vi "power supply newest.vi"() -> ()   [LabVIEW 2022 SP3]
uses:
  <vilib>/DAQmx/create/channels.llb/DAQmx Create Channel (AI-Voltage-Basic).vi
  <vilib>/DAQmx/read.llb/DAQmx Read (Analog DBL 1Chan 1Samp).vi
panel:
  in  "physical channels":tag
  out "temperature":dbl
  out "data":dbl format="%0.2f"
  in  "stop":bool
  in  "VISA resource name":refnum<visa-resource-name>
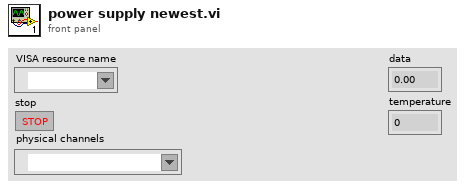
[diagram p1: front panel]
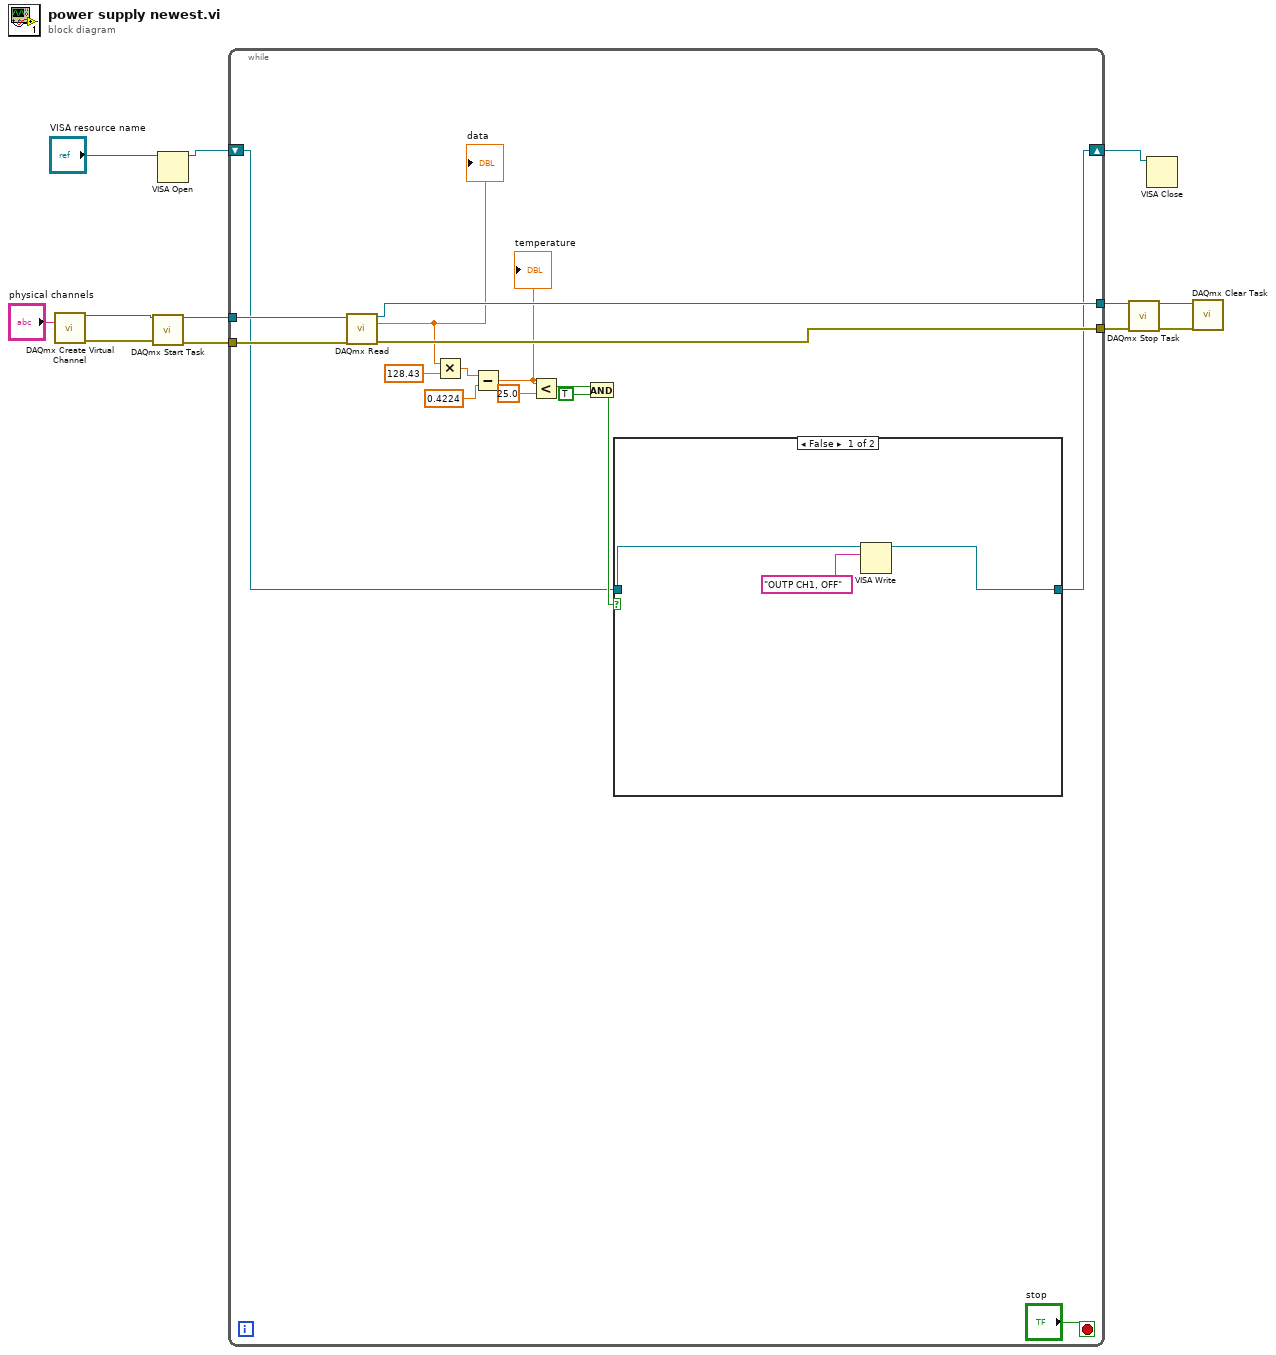
[diagram p0: block diagram]
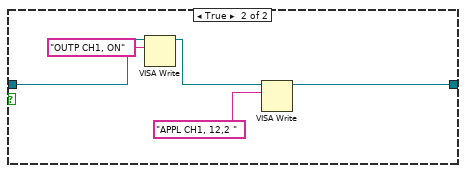
[diagram p2: hidden frame]
diagram:
  n1 = call-poly <vilib>:"DAQmx Create Virtual Channel.vi"("physical channels"="physical channels") -> ("task out"=w9:refnum<k21>, "error out"=w5:errorcluster)  [unwired: 13 in]
  n2 = call <vilib>:"DAQmx Start Task.vi"("task/channels in"=w9, "error in"=w5) -> ("task out"=w8:refnum<k21>, "error out"=w4:errorcluster)  [unwired: 12 in]
  n3 = VISA Open(VISA resource name="VISA resource name") -> (VISA resource name=w11:refnum<visa-resource-name>)  [unwired: 4 in, 1 out]
  n4 = while {
    shift-right: [w14] -> w10
    shift-left: w11 -> [w13]
    tunnel: w8 -> [w27]
    tunnel: w4 -> [w26]
    tunnel: [w25] -> w3
    tunnel: [w24] -> w2
    stop <- "stop" stop-if-true
    n5 = call-poly <vilib>:"DAQmx Read.vi"("task/channels in"=w27, "error in"=w26) -> ("task out"=w25:refnum<k21>, "data"=w22:dbl, "error out"=w24:errorcluster)  [unwired: 11 in]
    "data" <- w22
    n6 = Multiply(x=w22, y=128.43) -> (x*y=w23:dbl)
    n7 = Subtract(x=w23, y=0.4224 ("x*y")) -> (x-y=w19:dbl)
    "temperature" <- w19
    n8 = Less?(x=w19, y=25.0) -> (x < y?=w17:bool)
    n9 = And(x=w17, y=TRUE) -> (x .and. y?=w15:bool)
    n10 = case shown="False" w15 {
      tunnel: [w31 w36] -> w14
      tunnel: w13 -> [w30 w35]
      frame False {
        n11 = VISA Write(VISA resource name=w30, write buffer="OUTP CH1, OFF") -> (VISA resource name out=w31:refnum<visa-resource-name>)  [unwired: 1 in, 2 out]
      }
      frame True {
        n12 = VISA Write(VISA resource name=w35, write buffer="OUTP CH1, ON") -> (VISA resource name out=w34:refnum<visa-resource-name>)  [unwired: 1 in, 2 out]
        n13 = VISA Write(VISA resource name=w34, write buffer="APPL CH1, 12,2 ") -> (VISA resource name out=w36:refnum<visa-resource-name>)  [unwired: 1 in, 2 out]
      }
    }
  }
  n14 = call <vilib>:"DAQmx Stop Task.vi"("task/channels in"=w3, "error in"=w2) -> ("task out"=w7:refnum<k21>, "error out"=w6:errorcluster)  [unwired: 12 in]
  n15 = VISA Close(VISA resource name=w10) -> ()  [unwired: 1 in, 1 out]
  n16 = call <vilib>:"DAQmx Clear Task.vi"("task in"=w7, "error in"=w6) -> ()  [unwired: 13 in, 1 out]
